vi "connection_process.vi"(6 "timeout (ms)":i32=1000, 11 "TCPConnection":refnum<class "TCPConnection.lvclass">) -> ()   [LabVIEW 2013, in "MQTT Server.lvlib" / "TCPConnection.lvclass"]
uses:
  TCPConnection.lvclass
  TCPConnection.lvclass/TCPConnection.ctl
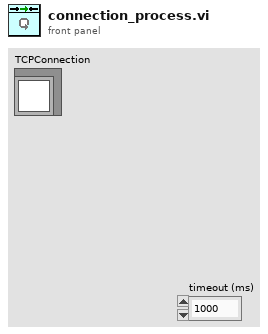
[diagram p1: front panel]
types:
  T1 = cluster{"connection ID":refnum<k5>, "error out":errorcluster}
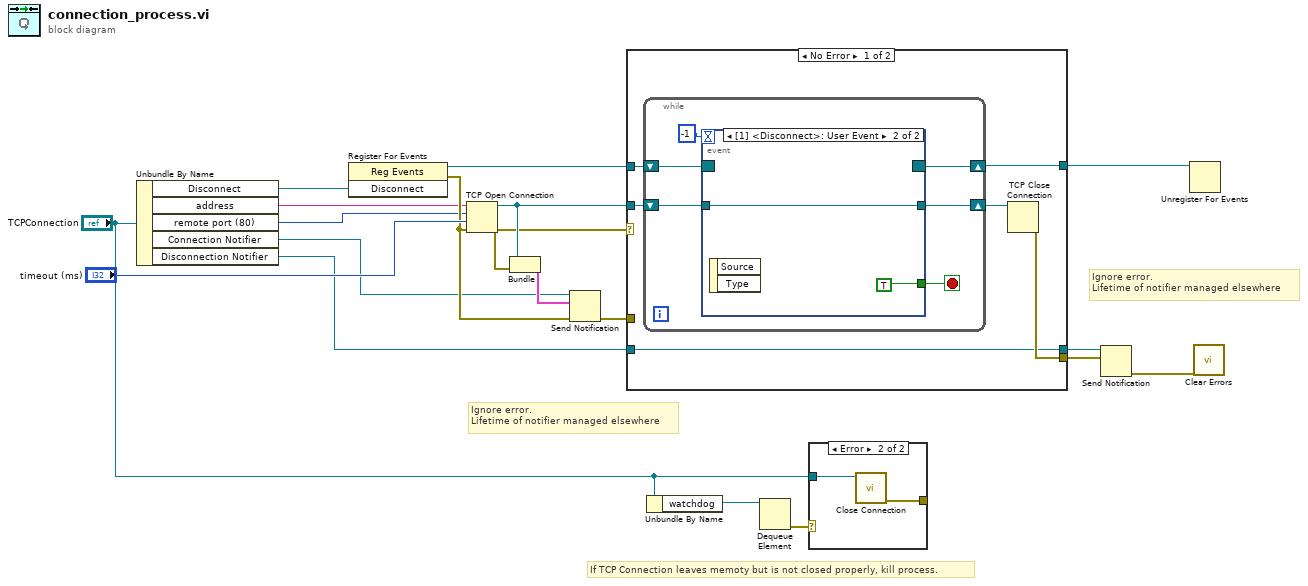
[diagram p0: block diagram]
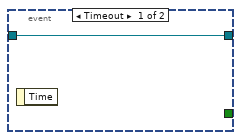
[diagram p3: hidden frame]
diagram:
  # "If TCP Connection leaves memoty but is not closed properly, kill process."
  # "Ignore error.\nLifetime of notifier managed elsewhere"
  # "Ignore error.\nLifetime of notifier managed elsewhere"
  n1 = Unbundle By Name("TCPConnection") -> ("Disconnect"=w11:refnum<user-event>, "address"=w9:string, "remote port (80)"=w8:u16, "Connection Notifier"=w10:refnum<notifier>, "Disconnection Notifier"=w4:refnum<notifier>)
  n2 = register-events(w11) -> (reference out=w15:refnum<event-registration>, error out=w14:errorcluster)  [unwired: 2 in]
  n3 = TCP Open Connection(address=w9, remote port or service name=w8, timeout ms (60000)="timeout (ms)", error in (no error)=w14) -> (connection ID=w17:refnum<k5>, error out=w13:errorcluster)  [unwired: 1 in]
  n4 = Bundle("connection ID"=w17, "error out"=w13) -> (w19:T1)  [unwired: 1 in]
  n5 = Send Notification(notification=w19, notifier=w10, error in (no error)=w14) -> (error out=w12:errorcluster)  [unwired: 1 out]
  n6 = case shown="No Error" w13 {
    selector: w13 -> [_ w36]
    tunnel: w17 -> [w25 _]
    tunnel: [w23 w37] -> w16
    tunnel: w15 -> [w22 w37]
    tunnel: w12 -> [_ _]
    tunnel: [w21 w36] -> w7
    tunnel: w4 -> [w20 w35]
    tunnel: [w20 w35] -> w6
    frame No Error {
      n7 = while {
        shift-right: [w29] -> w24
        shift-left: w25 -> [w30]
        shift-right: [w28] -> w23
        shift-left: w22 -> [w27]
        stop <- w26 stop-if-true
        n8 = event shown="[1] <Disconnect>: User Event" {
          selector: w27 -> [_ _]
          dyn-events: [_ _] -> w28
          timeout: -1 -> [_ _]
          tunnel: w30 -> [w32 w34]
          tunnel: [w32 w34] -> w29
          tunnel: [_ TRUE] -> w26
          event Timeout {
            n9 = event-data() -> ()  [unwired: 1 in, 1 out]
          }
          event User Event {
            n10 = event-data() -> ()  [unwired: 1 in, 2 out]
          }
        }
      }
      n11 = TCP Close Connection(connection ID=w24) -> (error out=w21:errorcluster)  [unwired: 2 in, 1 out]
    }
    frame Error {
    }
  }
  n12 = Unbundle By Name("TCPConnection") -> ("watchdog"=w3:refnum<queue>)
  n13 = Dequeue Element(queue=w3) -> (error out=w2:errorcluster)  [unwired: 2 in, 3 out]
  n14 = case shown="Error" w2 {
    tunnel: [_ w38] -> _
    tunnel: "TCPConnection" -> [_ w39]
    frame No Error {
    }
    frame Error {
      n15 = call-dynamic "Close Connection.vi"("TCPConnection in"=w39) -> ("error out"=w38:errorcluster)  [unwired: 9 in, 1 out]
    }
  }
  n16 = Send Notification(notification=w7, notifier=w6) -> (error out=w5:errorcluster)  [unwired: 1 in, 1 out]
  n17 = Unregister For Events(event registration refnum=w16) -> ()  [unwired: 1 in, 1 out]
  n18 = call <vilib>:"Clear Errors.vi"("error in (no error)"=w5) -> ()  [unwired: 6 in, 1 out]
